vi "DestroyIcon.vi"(4 "error in (no error)":errorcluster, 7 "hIcon":i32) -> (0 "error out":errorcluster)   [LabVIEW 2011]
uses:
  user32.dll
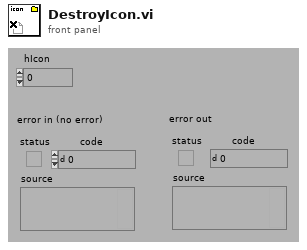
[diagram p1: front panel]
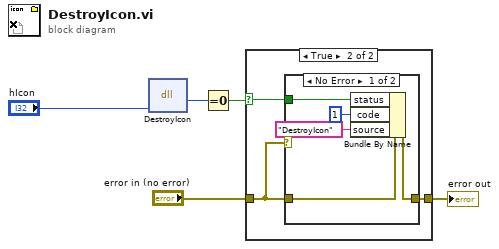
[diagram p0: block diagram]
diagram:
  n1 = dll-call lib="User32.dll" fn="DestroyIcon"("hIcon"="hIcon") -> (w4:i32)  [unwired: 4 in, 2 out]
  n2 = Equal To 0?(x=w4) -> (x = 0?=w3:bool)
  n3 = case shown="True" w3 {
    selector: w3 -> [_ w9]
    tunnel: "error in (no error)" -> [w6 w7]
    tunnel: [w6 w8] -> w1
    frame False {
    }
    frame True {
      n4 = case shown="No Error" w7 {
        tunnel: w7 -> [w14 w15]
        tunnel: w9 -> [w13 _]
        tunnel: [w12 w15] -> w8
        frame No Error {
          n5 = Bundle By Name(cluster=w14, "status"=w13, "code"=1, "source"="DestroyIcon") -> (w12:errorcluster)
        }
        frame Error {
        }
      }
    }
  }
  "error out" <- w1
